vi "Is Null.vi"(11 "Config Element in":refnum<class "Config Element.lvclass">) -> (3 "Null":bool)   [LabVIEW 2020, in "CDM-Config.lvlib" / "Config Element.lvclass"]
doc: "Returns true if the class is not a valid element instance."
uses:
  Config Element.lvclass
  Meta Data.ctl
  CDM-Config.lvlib
  Node Info.ctl
  Ref Data.ctl
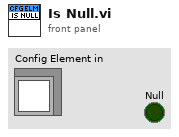
[diagram p1: front panel]
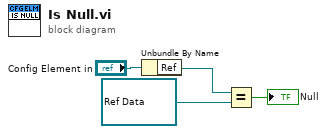
[diagram p0: block diagram]
diagram:
  n1 = Unbundle By Name("Config Element in") -> ("Ref"=w2:refnum<data-value>)
  n2 = Equal?(x=w2, y=refnum<data-value> refnum) -> (x = y?=→"Null":bool)
